vi "Receive User Menu Selection Msg.vi"(8 "error in (no error)":errorcluster, 10 "UserMenuSelectionMsg":refnum<class "UserMenuSelectionMsg.lvclass">, 11 "ConcreteViewModel in":refnum<class "ConcreteViewModel.lvclass">) -> (0 "error out":errorcluster, 3 "ConcreteViewModel out":refnum<class "ConcreteViewModel.lvclass">)   [LabVIEW 2015, in "TopLevelApplication.lvlib" / "ConcreteViewModel.lvclass"]
doc: "<License>\nCopyright © 2017 Composed Systems, LLC | All rights reserved\nwww.composed.io\n\nAuthor: Ethan Stern <ethan.stern@composed.io>\n\nThis software is provided \"AS IS\" WITHOUT WARRANTIES, either express or implied, AND IS FOR EDUCATIONAL PURPOSES ONLY.\n</License>"
uses:
  ConcreteViewModel.lvclass
  Framework/AutoRegistration/ActorAutoRegistration Messages/UserMenuSelectionMsg/UserMenuSelectionMsg.lvclass
  Dialog Box Implementations/OneButtonDialogBox/OneButtonDialogBox.lvclass
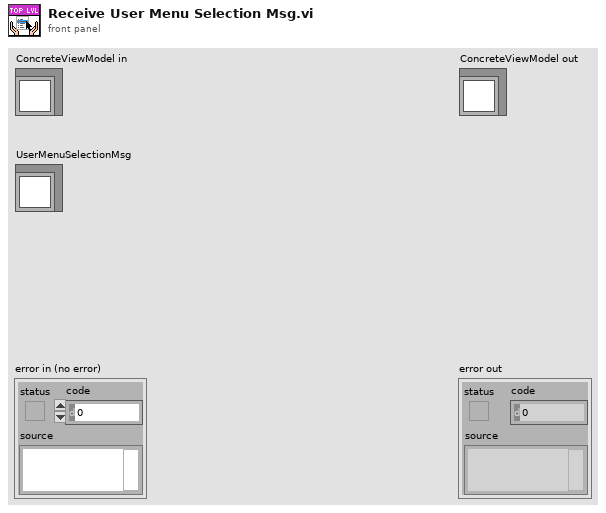
[diagram p1: front panel]
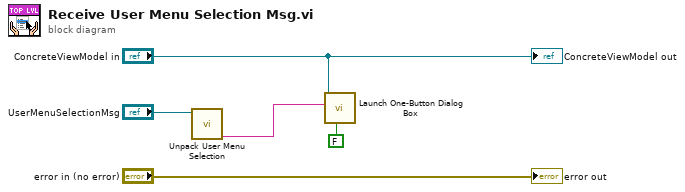
[diagram p0: block diagram]
diagram:
  n1 = call-dynamic "Unpack User Menu Selection.vi"("UserMenuSelectionMsg In"="UserMenuSelectionMsg") -> ("Item Path"=w2:string)  [unwired: 7 in, 3 out]
  n2 = call "Launch One-Button Dialog Box.vi"("Modal? (T)"=FALSE, "Message Text"=w2, "Dialog Launcher"="ConcreteViewModel in") -> ()  [unwired: 8 in, 1 out]
  "error out" <- "error in (no error)"
  "ConcreteViewModel out" <- "ConcreteViewModel in"
